vi "Periodic Tasks.vi"() -> ()   [LabVIEW 2011]
doc: "This VI runs in parallel to other tasks. It can contain as many user-defined periodic loops as you need. These can carry out PID or other sorts of timed response."
uses:
  <vilib>/Rock Robotics/SystemInterfaces/Utilities/FPGA_UtilitiesLED State.ctl
  <vilib>/Rock Robotics/SystemInterfaces/Utilities/FPGA_UtilitiesLED Source.ctl
  Robot Global Data.vi
  <vilib>/Rock Robotics/WPI/Relay/WPI_RelayValue.ctl
panel:
  in  "Speed of Harvester":dbl
  in  "Speed of Conveyor":dbl
  out "Right Rate":dbl
  out "error out 4":errorcluster
  out "Right Direction":bool
  out "Right Distance":dbl
  out "Distance 2":dbl
  out "Direction 2":bool
  out "error out 3":errorcluster
  out "Rate 2":dbl
  out "Left Rate":dbl
  out "error out 2":errorcluster
  out "I2C":bool
  out "Angular Rate":dbl
  out "Angle":dbl
  out "Left Direction":bool
  out "Left Distance":dbl
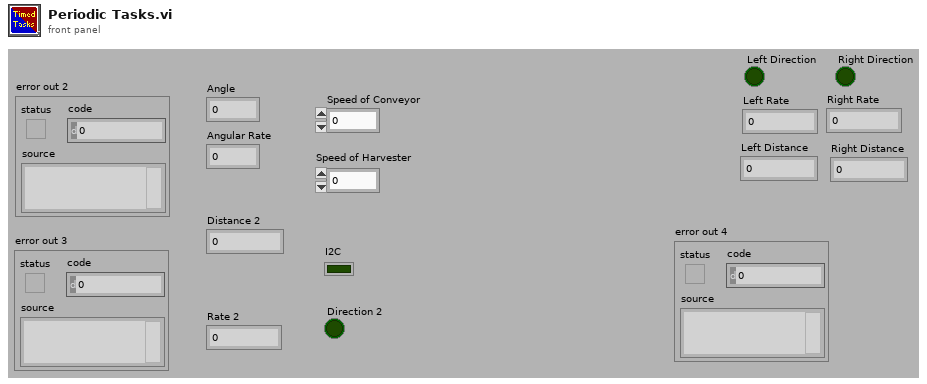
[diagram p1: front panel]
types:
  T1 = typedef "WPI_RelayValue.ctl" = enum16{"Off", "On", "Forward", "Reverse"}
  T2 = typedef "WPI_AnalogChannelDevRef.ctl" = cluster{"DevStatus":errorcluster, "Analog Module":T3, "Analog Channel":T4}
  T3 = typedef "FPGA_TypedefAnalogModule.ctl" = enum16{"Analog Module 1", "Analog Module 2"}
  T4 = typedef "FPGA_AIChannel.ctl" = enum8{"AI 1", "AI 2", "AI 3", "AI 4", "AI 5", "AI 6", "AI 7", "AI 8", "Invalid"}
  T5 = typedef "WPI_EncoderDevRef.ctl" = cluster{"DevStatus":errorcluster, "EncoderIndex":T6, "CounterIndex":T7, "DistancePerCount":dbl, "Decoding Type":T8}
  T6 = typedef "FPGA_EncoderIdx.ctl" = enum8{"Enc 0", "Enc 1", "Enc 2", "Enc 3", "Invalid"}
  T7 = typedef "FPGA_CounterCtrSystemIndex.ctl" = enum8{"Ctr 0", "Ctr 1", "Ctr 2", "Ctr 3", "Ctr 4", "Ctr 5", "Ctr 6", "Ctr 7", "Invalid"}
  T8 = typedef "WPI_EncoderType.ctl" = enum16{"1x", "2x", "4x"}
  T9 = typedef "WPI_RelayDevRef.ctl" = cluster{"DevStatus":errorcluster, "Relay Channel":T10, "Digital Module":T11, "Relay Direction":T12}
  T10 = typedef "FPGA_DIORelayChannel.ctl" = enum8{"Relay 1", "Relay 2", "Relay 3", "Relay 4", "Relay 5", "Relay 6", "Relay 7", "Relay 8", "Invalid"}
  T11 = typedef "FPGA_TypedefDigitalModule.ctl" = enum16{"Digital Module 1", "Digital Module 2"}
  T12 = typedef "WPI_RelayDirection.ctl" = enum16{"Both directions", "Forward only", "Reverse only"}
  T13 = typedef "WPI_GyroDevRef.ctl" = cluster{"DevStatus":errorcluster, "Analog Module":T3, "Analog Channel":T4, "Offset":dbl, "Gain (VoltsPerDegree/Second)":dbl}
  T14 = cluster{"Driver Station Digital Output (1-8)[0]":bool, "Driver Station Digital Output (1-8)[1]":bool, "Driver Station Digital Output (1-8)[2]":bool, "Driver Station Digital Output (1-8)[3]":bool, "Driver Station Digital Output (1-8)[4]":bool, "Driver Station Digital Output (1-8)[5]":bool, "Driver Station Digital Output (1-8)[6]":bool, "Driver Station Digital Output (1-8)[7]":bool, "Driver Station Digital Output (1-8)[8]":bool}
  T15 = typedef "FPGA_UtilitiesLED State.ctl" = enum16{"Off", "On", "Toggle"}
  T16 = typedef "FPGA_UtilitiesLED Source.ctl" = enum16{"User LED", "FPGA LED"}
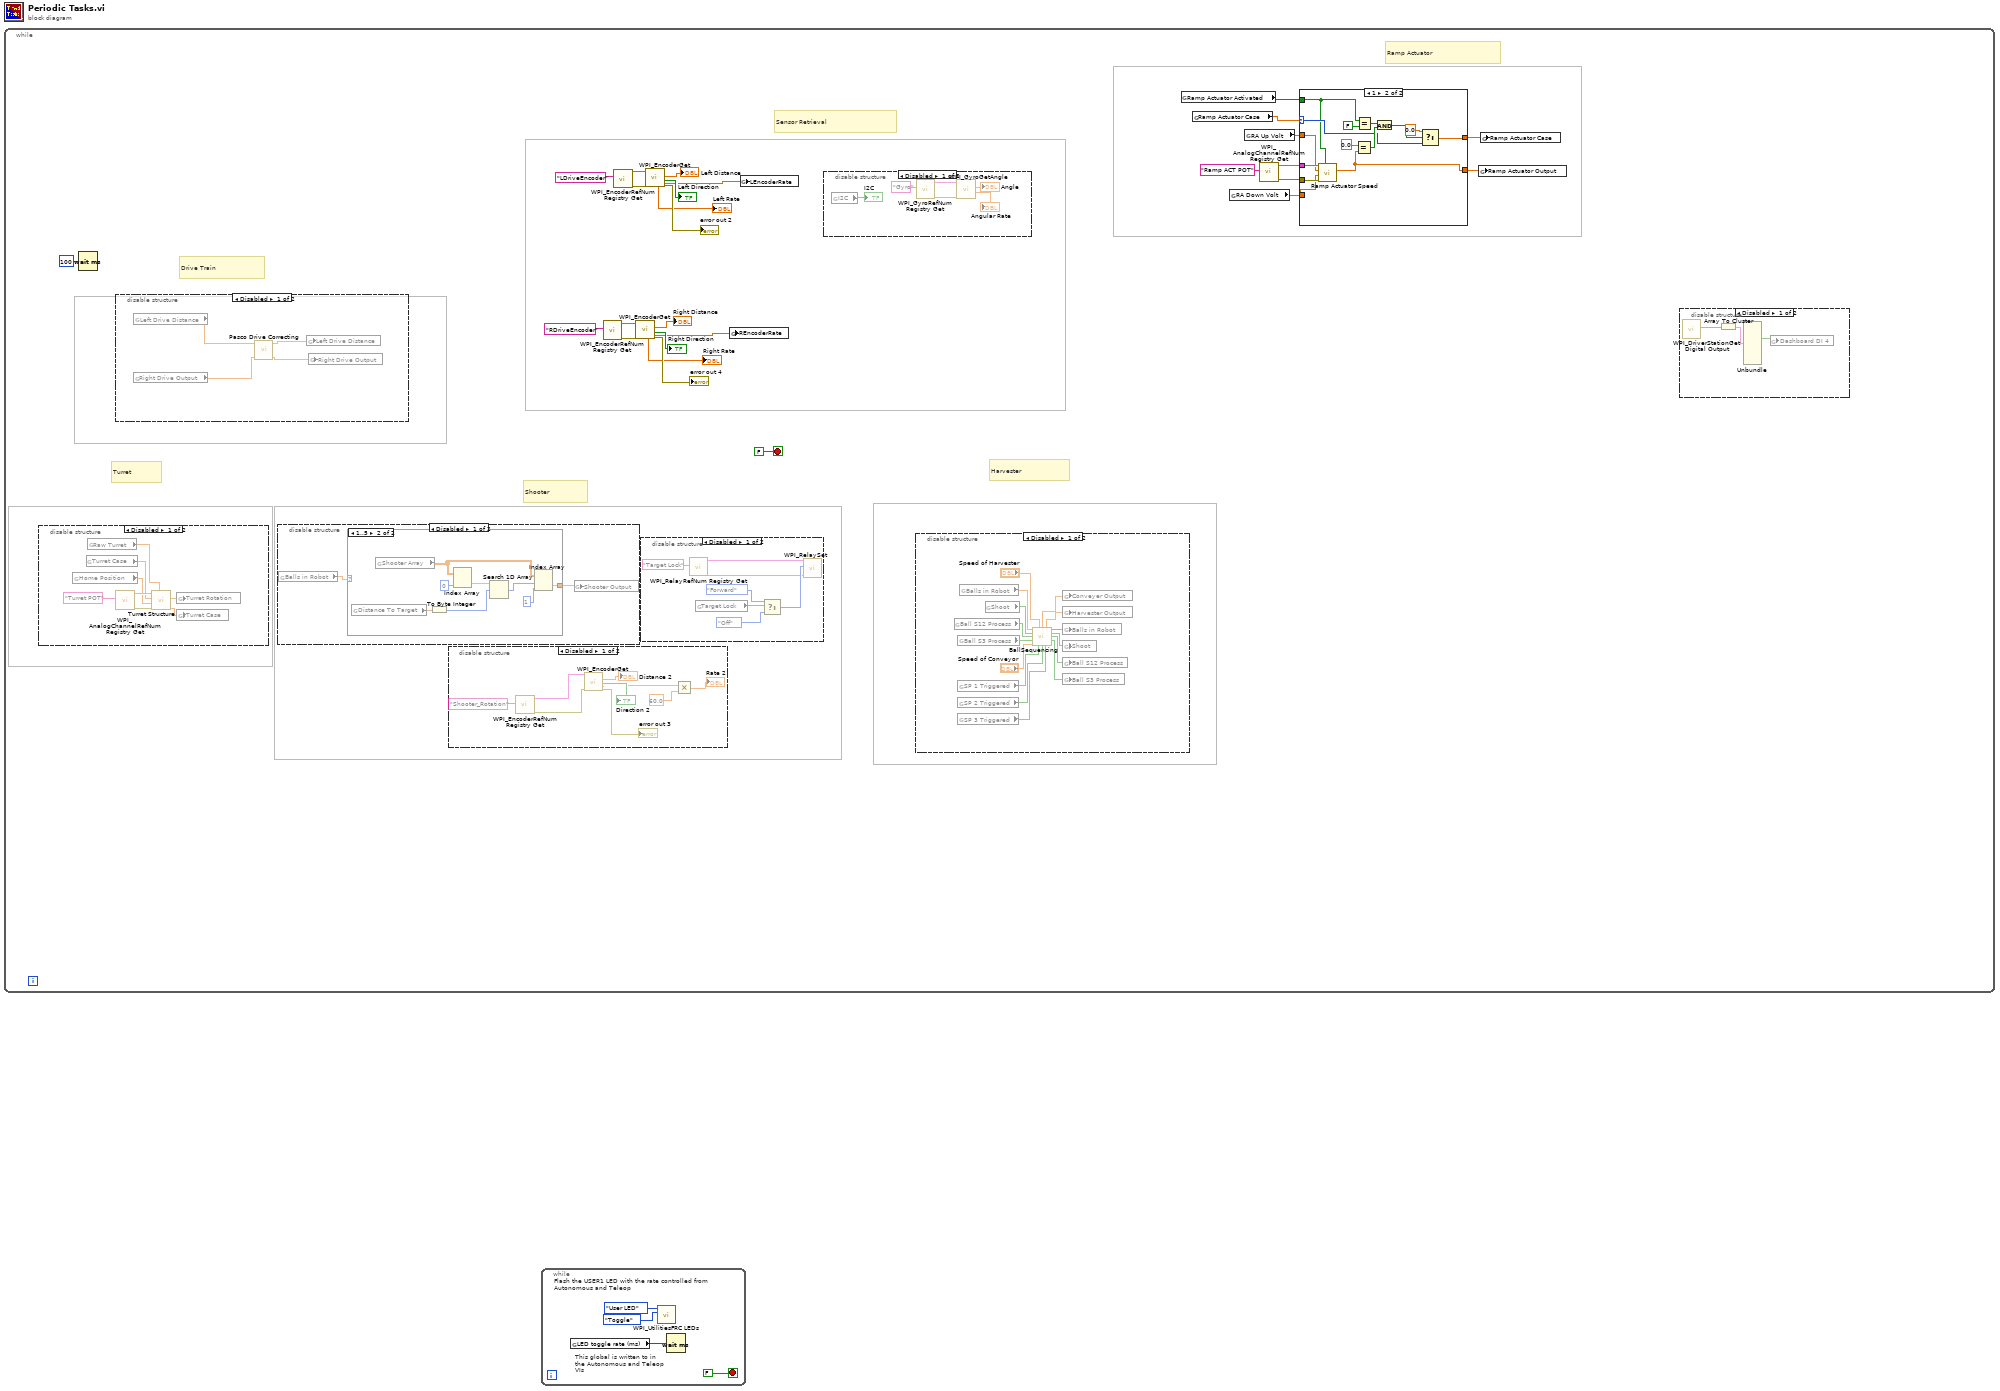
[diagram p0: block diagram]
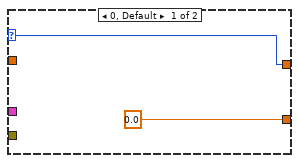
[diagram p2: hidden frame]
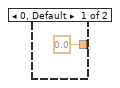
[diagram p3: hidden frame]
diagram:
  n1 = while {
    stop <- FALSE stop-if-true
    # "Harvester"
    # "Shooter"
    # "Sensor Retrieval"
    # "Turret"
    # "Drive Train"
    # "Ramp Actuator"
    n2 = disable-structure shown="Disabled" {
      frame Disabled {
        n3 = global read "Robot Global Data.vi" "Home Position"() -> (w78:dbl)
        n4 = global read "Robot Global Data.vi" "Turret Case"() -> (w79:dbl)
        n5 = global read "Robot Global Data.vi" "Raw Turret"() -> (w77:dbl)
        n6 = call <vilib>:"WPI_AnalogChannelRefNum Registry Get.vi"("refnum name"="Turret POT") -> ("error out"=w80:errorcluster, "AIDeviceRef"=w81:T2)  [unwired: 9 in]
        n7 = call "Turret Structure.vi"("Raw Turret"=w77, "error in (no error)"=w80, "Home postion"=w78, "Turret Case"=w79, "AIDeviceRef"=w81) -> ("Turret Case Output"=w75:dbl, "Turret Output"=w76:dbl)  [unwired: 5 in]
        n8 = global write "Robot Global Data.vi" "Turret Rotation"(w76) -> ()
        n9 = global write "Robot Global Data.vi" "Turret Case"(w75) -> ()
      }
      frame Enabled {
      }
    }
    n10 = Wait (ms)(milliseconds to wait=u32 100) -> ()  [unwired: 1 out]
    n11 = disable-structure shown="Disabled" {
      frame Disabled {
        n12 = global read "Robot Global Data.vi" "Right Drive Output"() -> (w85:dbl)
        n13 = global read "Robot Global Data.vi" "Left Drive Distance"() -> (w86:dbl)
        n14 = call "Pasco Drive Correcting.vi"("RightDriveOutput"=w85, "LeftDriveOutput"=w86) -> ("RightDriveOutput"=w83:dbl, "LeftDriveOutput"=w84:dbl)  [unwired: 8 in]
        n15 = global write "Robot Global Data.vi" "Left Drive Distance"(w84) -> ()
        n16 = global write "Robot Global Data.vi" "Right Drive Output"(w83) -> ()
      }
      frame Enabled {
      }
    }
    n17 = disable-structure shown="Disabled" {
      frame Disabled {
        n18 = global read "Robot Global Data.vi" "Balls in Robot"() -> (w42:dbl)
        n19 = case shown="1..5" w42 {
          tunnel: [0.0 w45] -> w43
          frame 0, Default {
          }
          frame 1..5 {
            n20 = global read "Robot Global Data.vi" "Distance To Target"() -> (w50:dbl)
            n21 = global read "Robot Global Data.vi" "Shooter Array"() -> (w48:dbl[][])
            n22 = To Byte Integer(number=w50) -> (8bit integer=w49:i8)
            n23 = Index Array(array=w48, index (col)=0 ("disabled index (col)")) -> (element=w51:dbl[])  [unwired: 1 in]
            n24 = Search 1D Array(1D array=w51, element=w49) -> (index of element=w47:i32)  [unwired: 1 in]
            n25 = Index Array(array=w48, index (row)=w47, index (col)=1 ("disabled index (col)")) -> (element=w45:dbl)
          }
        }
        n26 = global write "Robot Global Data.vi" "Shooter Output"(w43) -> ()
      }
      frame Enabled {
      }
    }
    n27 = disable-structure shown="Disabled" {
      frame Disabled {
        n28 = call <vilib>:"WPI_EncoderRefNum Registry Get.vi"("refnum name"="Shooter_Rotation") -> ("error out"=w96:errorcluster, "EncoderDevRef"=w97:T5)  [unwired: 9 in]
        n29 = call <vilib>:"WPI_EncoderGet.vi"("error in (no error)"=w96, "EncoderDevRef"=w97) -> ("error out"=→"error out 3":errorcluster, "Direction"=→"Direction 2":bool, "Distance"=→"Distance 2":dbl, "Rate"=w100:dbl)  [unwired: 4 in, 2 out]
        n30 = Multiply(x=w100, y=60.0) -> (x*y=→"Rate 2":dbl)
      }
      frame Enabled {
      }
    }
    n31 = call <vilib>:"WPI_EncoderRefNum Registry Get.vi"("refnum name"="RDriveEncoder") -> ("error out"=w14:errorcluster, "EncoderDevRef"=w13:T5)  [unwired: 9 in]
    n32 = call <vilib>:"WPI_EncoderRefNum Registry Get.vi"("refnum name"="LDriveEncoder") -> ("error out"=w21:errorcluster, "EncoderDevRef"=w20:T5)  [unwired: 9 in]
    n33 = call <vilib>:"WPI_EncoderGet.vi"("error in (no error)"=w14, "EncoderDevRef"=w13) -> ("error out"=→"error out 4":errorcluster, "Direction"=→"Right Direction":bool, "Distance"=→"Right Distance":dbl, "Rate"=w10:dbl)  [unwired: 4 in, 2 out]
    "Right Rate" <- w10
    n34 = disable-structure shown="Disabled" {
      frame Disabled {
        n35 = call <vilib>:"WPI_RelayRefNum Registry Get.vi"("refnum name"="Target Lock") -> ("error out"=w68:errorcluster, "RelayDevRef"=w69:T9)  [unwired: 9 in]
        n36 = global read "Robot Global Data.vi" "Target Lock"() -> (w74:bool)
        n37 = Select(t=WPI_RelayValue."Forward" ("RelayValue"), s=w74, f=WPI_RelayValue."Off" ("RelayValue")) -> (s? t:f=w71:T1)
        n38 = call <vilib>:"WPI_RelaySet.vi"("error in (no error)"=w68, "RelayValue"=w71, "RelayDevRef"=w69) -> ()  [unwired: 7 in, 2 out]
      }
      frame Enabled {
      }
    }
    n39 = call <vilib>:"WPI_EncoderGet.vi"("error in (no error)"=w21, "EncoderDevRef"=w20) -> ("error out"=→"error out 2":errorcluster, "Direction"=→"Left Direction":bool, "Distance"=→"Left Distance":dbl, "Rate"=w17:dbl)  [unwired: 4 in, 2 out]
    "Left Rate" <- w17
    n40 = global write "Robot Global Data.vi" "REncoderRate"(w10) -> ()
    n41 = global write "Robot Global Data.vi" "LEncoderRate"(w17) -> ()
    n42 = disable-structure shown="Disabled" {
      frame Disabled {
        n43 = global read "Robot Global Data.vi" "I2C"() -> (→"I2C":bool)
        n44 = call <vilib>:"WPI_GyroRefNum Registry Get.vi"("refnum name"="Gyro") -> ("error out"=w94:errorcluster, "GyroDevRef"=w95:T13)  [unwired: 9 in]
        n45 = call <vilib>:"WPI_GyroGetAngle.vi"("error in (no error)"=w94, "GyroDevRef"=w95) -> ("Angular Rate"=→"Angular Rate":dbl, "Angle"=→"Angle":dbl)  [unwired: 6 in, 2 out]
      }
      frame Enabled {
      }
    }
    n46 = disable-structure shown="Disabled" {
      frame Disabled {
        n47 = global read "Robot Global Data.vi" "Ball S12 Process"() -> (w54:bool)
        n48 = global read "Robot Global Data.vi" "Ball S3 Process"() -> (w53:bool)
        n49 = global read "Robot Global Data.vi" "SP 1 Triggered"() -> (w61:bool)
        n50 = global read "Robot Global Data.vi" "SP 2 Triggered"() -> (w62:bool)
        n51 = global read "Robot Global Data.vi" "SP 3 Triggered"() -> (w63:bool)
        n52 = global read "Robot Global Data.vi" "Balls in Robot"() -> (w56:dbl)
        n53 = global read "Robot Global Data.vi" "Shoot"() -> (w55:bool)
        n54 = call "BallSequencing.vi"("Balls In Robot"=w56, "Speed of Harvester"="Speed of Harvester", "Shoot"=w55, "Ball S12 Process"=w54, "Ball S3 Process"=w53, "Speed of Conveyor"="Speed of Conveyor", "SP 1 Triggered"=w61, "SP 2 Triggered"=w62, "SP 3 Triggered"=w63) -> ("Conveyer Output"=w57:dbl, "Harvester Output"=w58:dbl, "Balls In Robot Output"=w67:i32, "Shoot Output"=w66:bool, "Ball S12 Process Output"=w65:bool, "Ball S3 Process Output"=w64:bool)  [unwired: 1 in]
        n55 = global write "Robot Global Data.vi" "Conveyer Output"(w57) -> ()
        n56 = global write "Robot Global Data.vi" "Harvester Output"(w58) -> ()
        n57 = global write "Robot Global Data.vi" "Balls in Robot"(w67) -> ()
        n58 = global write "Robot Global Data.vi" "Shoot"(w66) -> ()
        n59 = global write "Robot Global Data.vi" "Ball S12 Process"(w65) -> ()
        n60 = global write "Robot Global Data.vi" "Ball S3 Process"(w64) -> ()
      }
      frame Enabled {
      }
    }
    n61 = global read "Robot Global Data.vi" "Ramp Actuator Activated"() -> (w1:bool)
    n62 = global read "Robot Global Data.vi" "Ramp Actuator Case"() -> (w3:dbl)
    n63 = global read "Robot Global Data.vi" "RA Down Volt"() -> (w6:dbl)
    n64 = global read "Robot Global Data.vi" "RA Up Volt"() -> (w5:dbl)
    n65 = call <vilib>:"WPI_AnalogChannelRefNum Registry Get.vi"("refnum name"="Ramp ACT POT") -> ("error out"=w7:errorcluster, "AIDeviceRef"=w8:T2)  [unwired: 9 in]
    n66 = case shown="1" w3 {
      selector: w3 -> [w26 w30]
      tunnel: w8 -> [_ w41]
      tunnel: w7 -> [_ w40]
      tunnel: w6 -> [_ w39]
      tunnel: w5 -> [_ w38]
      tunnel: [0.0 ("Ramp Actuator Ouput") w29] -> w4
      tunnel: w1 -> [_ w28]
      tunnel: [w26 w31] -> w2
      frame 0, Default {
      }
      frame 1 {
        n67 = call "Ramp Actuator Speed.vi"("Up to Down"=w28, "error in (no error)"=w40, "RA Down Volt"=w39, "RA Up Volt"=w38, "AIDeviceRef"=w41) -> ("Ramp Actuator Ouput"=w29:dbl)  [unwired: 6 in]
        n68 = Equal?(x=0.0, y=w29) -> (x = y?=w36:bool)
        n69 = Equal?(x=w28, y=FALSE) -> (x = y?=w35:bool)
        n70 = And(x=w35, y=w36) -> (x .and. y?=w33:bool)
        n71 = Select(t=0.0, s=w33, f=w30) -> (s? t:f=w31:dbl)
      }
    }
    n72 = global write "Robot Global Data.vi" "Ramp Actuator Output"(w4) -> ()
    n73 = global write "Robot Global Data.vi" "Ramp Actuator Case"(w2) -> ()
    n74 = disable-structure shown="Disabled" {
      frame Disabled {
        n75 = call <vilib>:"WPI_DriverStationGet Digital Output.vi"() -> ("Driver Station Digital Output (1-8)"=w89:bool[])  [unwired: 10 in, 1 out]
        n76 = Array To Cluster(array=w89) -> (cluster=w88:T14)
        n77 = Unbundle(w88) -> ("Driver Station Digital Output (1-8)[3]"=w87:bool)  [unwired: 8 out]
        n78 = global write "Robot Global Data.vi" "Dashboard DI 4"(w87) -> ()
      }
      frame Enabled {
      }
    }
  }
  n79 = while {
    stop <- FALSE stop-if-true
    # "This global is written to in the Autonomous and Teleop VIs"
    # "Flash the USER1 LED with the rate controlled from Autonomous and Teleop"
    n80 = global read "Robot Global Data.vi" "LED toggle rate (ms)"() -> (w105:u32)
    n81 = call <vilib>:"WPI_UtilitiesFRC LEDs.vi"("State"=FPGA_UtilitiesLED_State."Toggle", "LED Type"=FPGA_UtilitiesLED_Source."User LED") -> ()  [unwired: 1 in, 9 out]
    n82 = Wait (ms)(milliseconds to wait=w105) -> ()  [unwired: 1 out]
  }
